vi "get images.vi"(8 "error in (no error)":errorcluster, 11 "EnchantedRoom in":refnum<class "EnchantedRoom.lvclass">) -> (0 "error out":errorcluster, 2 "images":T1[](array[typedef]), 3 "EnchantedRoom out":refnum<class "EnchantedRoom.lvclass">)   [LabVIEW 2016, in "EnchantedRoom.lvclass"]
uses:
  EnchantedRoom.lvclass
  C:/github/LVOOP-creational-patterns/Maze-Classes/src/Base/Room/Room.lvclass
  <vilib>/picture/picture.llb/imagedata.ctl
  Base/Room/Room.lvclass
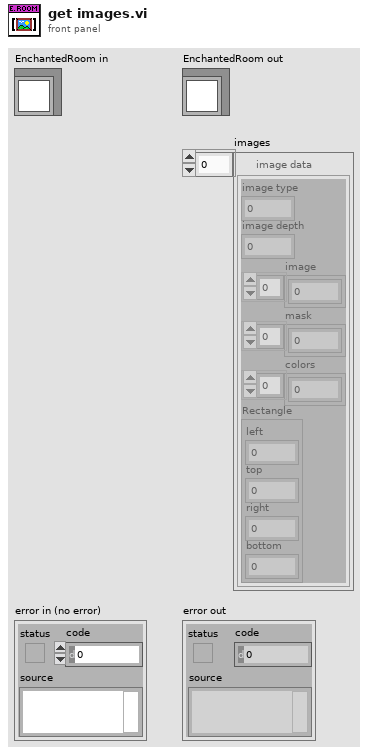
[diagram p1: front panel]
types:
  T1 = typedef "imagedata.ctl" = cluster{"image type":i32, "image depth":i32, "image":u8[], "mask":u8[], "colors":u32[], "Rectangle":cluster{"left":i16, "top":i16, "right":i16, "bottom":i16}}
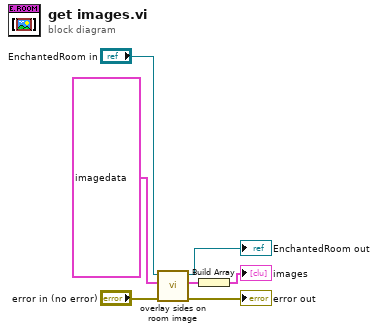
[diagram p0: block diagram]
diagram:
  n1 = call "overlay sides on room image.vi"("error in (no error)"="error in (no error)", "image data in"=T1 {"image type"=0, "image depth"=32, "image"=array[36864 elements], "mask"=array[1152 elements], "colors"=[], "Rectangle"={"left"=0, "top"=0, "right"=96, "bottom"=96}} ("image data"), "Room in"="EnchantedRoom in") -> ("error out"=→"error out":errorcluster, "image data  out"=w4:T1, "Room out"=→"EnchantedRoom out":refnum<class "EnchantedRoom.lvclass">)  [unwired: 6 in]
  n2 = Build Array(w4) -> (→"images":T1[])
